vi "GetParam.vi"(8 "error in (no error)":errorcluster caption="entrée d'erreur (pas d'erreur)", 11 "add_dummy_feature.lvclass":refnum<class "add_dummy_feature.lvclass">) -> (0 "error out":errorcluster caption="sortie d'erreur", 2 "add_dummy_feature":cluster{"value":dbl}={"value"=1.0}, 3 "add_dummy_feature.lvclass":refnum<class "add_dummy_feature.lvclass">)   [LabVIEW 2020, in "add_dummy_feature.lvclass"]
doc: "Get Parameters"
uses:
  add_dummy_feature.lvclass
  add_dummy_feature.lvclass/add_dummy_feature.ctl
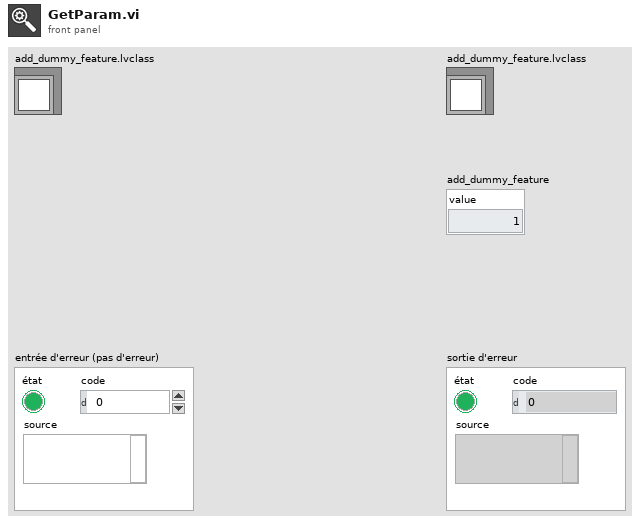
[diagram p1: front panel]
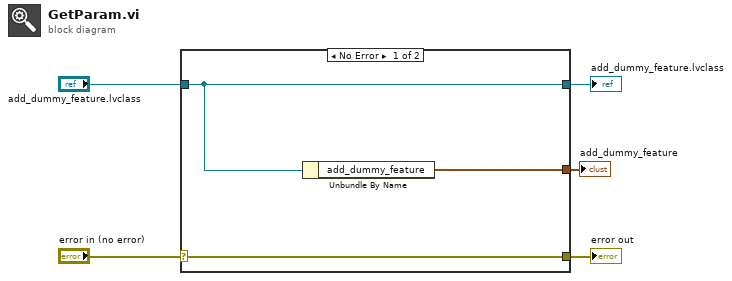
[diagram p0: block diagram]
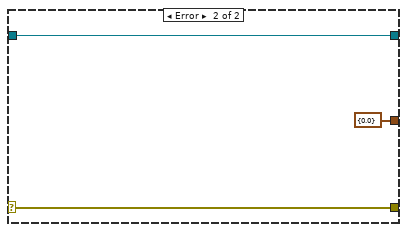
[diagram p2: hidden frame]
diagram:
  n1 = case shown="No Error" "error in (no error)" {
    selector: "error in (no error)" -> [w8 w10]
    tunnel: [w8 w10] -> w4
    tunnel: [w7 w11] -> w2
    tunnel: "add_dummy_feature.lvclass" -> [w7 w11]
    tunnel: [w6 cluster{"value":dbl} {"value"=0.0} ("add_dummy_feature")] -> w1
    frame No Error {
      n2 = Unbundle By Name(w7) -> ("add_dummy_feature"=w6:cluster{"value":dbl})
    }
    frame Error {
    }
  }
  "error out" <- w4
  "add_dummy_feature.lvclass" <- w2
  "add_dummy_feature" <- w1
